vi "Keith2probeSub.vi"(1 "GPIB Address":string) -> (0 "Numeric":dbl)   [LabVIEW 2017]
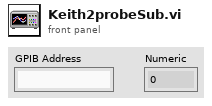
[diagram p1: front panel]
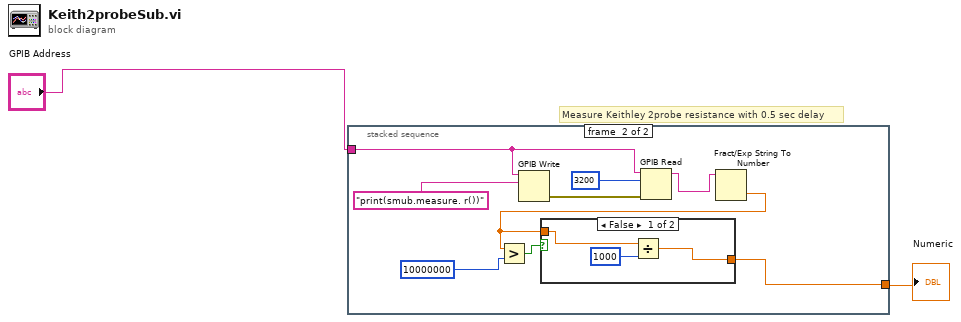
[diagram p0: block diagram]
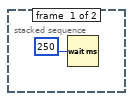
[diagram p2: hidden frame]
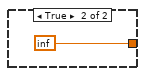
[diagram p3: hidden frame]
diagram:
  # "Measure Keithley 2probe resistance with 0.5 sec delay"
  n1 = stacked-sequence {
    tunnel: "GPIB Address" -> [_ w8]
    tunnel: [_ w4] -> w2
    frame #0 {
      n2 = Wait (ms)(milliseconds to wait=250) -> ()  [unwired: 1 out]
    }
    frame #1 {
      n3 = GPIB Write(0:w8, 1:"print(smub.measure. r())") -> (6:w9:errorcluster)  [unwired: 3 in, 1 out]
      n4 = GPIB Read(0:w8, 1:3200, 3:w9) -> (5:w12:string)  [unwired: 2 in, 2 out]
      n5 = Fract/Exp String To Number(string=w12) -> (number=w5:dbl)  [unwired: 3 in, 1 out]
      n6 = Greater?(x=w5, y=10000000) -> (0:w7:bool)
      n7 = case shown="False" w7 {
        tunnel: [w14 inf] -> w4
        tunnel: w5 -> [w15 _]
        frame False {
          n8 = Divide(x=w15, y=1000) -> (x/y=w14:dbl)
        }
        frame True {
        }
      }
    }
  }
  "Numeric" <- w2
